vi "VISA Query.vi"(4 "VISA Timeout (0ms=Unchanged)":u32, 6 "Read Delay (0ms)":u32, 8 "error in (no error)":errorcluster, 9 "Bytes to Read (0=No read)":u32, 10 "Write (\"\"=No write)":string, 11 "VISA in":refnum<visa-resource-name>) -> (0 "error out":errorcluster, 2 "Read":string, 3 "VISA out":refnum<visa-resource-name>)   [LabVIEW 2018]
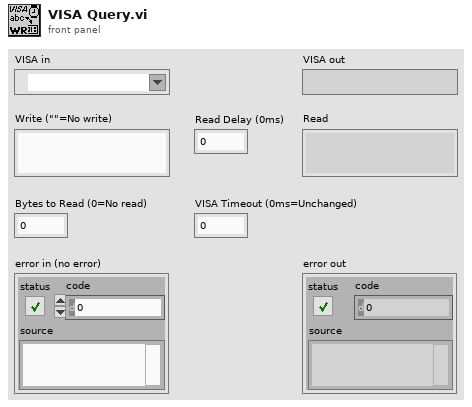
[diagram p1: front panel]
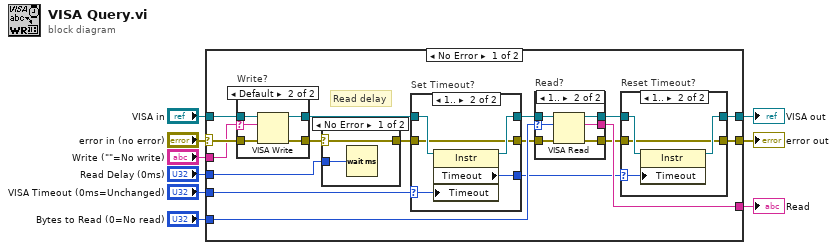
[diagram p0: block diagram]
diagram:
  n1 = case shown="No Error" "error in (no error)" {
    selector: "error in (no error)" -> [w26 w59]
    tunnel: "VISA in" -> [w25 w58]
    tunnel: "Write (\"\"=No write)" -> [w24 _]
    tunnel: "Bytes to Read (0=No read)" -> [w23 _]
    tunnel: [w22 _] -> w5
    tunnel: "Read Delay (0ms)" -> [w21 _]
    tunnel: "VISA Timeout (0ms=Unchanged)" -> [w17 _]
    tunnel: [w15 w58] -> w2
    tunnel: [w11 w59] -> w1
    frame No Error {
      # "Read delay"
      n2 = case "Write?" shown="Default" w24 {
        selector: w24 -> [_ w32]
        tunnel: w26 -> [w30 w36]
        tunnel: [w30 w35] -> w20
        tunnel: w25 -> [w31 w34]
        tunnel: [w31 w33] -> w19
        frame "" {
        }
        frame Default {
          n3 = VISA Write(VISA resource name=w34, write buffer=w32, error in (no error)=w36) -> (VISA resource name out=w33:refnum<visa-resource-name>, error out=w35:errorcluster)  [unwired: 1 out]
        }
      }
      n4 = case shown="No Error" w20 {
        selector: w20 -> [w27 w29]
        tunnel: w21 -> [w28 _]
        tunnel: [w27 w29] -> w12
        frame No Error {
          n5 = Wait (ms)(milliseconds to wait=w28) -> ()  [unwired: 1 out]
        }
        frame Error {
        }
      }
      n6 = case "Set Timeout?" shown="1.." w17 {
        selector: w17 -> [_ w41]
        tunnel: w19 -> [w38 w43]
        tunnel: [w38 w42] -> w18
        tunnel: [_ w40] -> w14
        tunnel: [w37 w39] -> w13
        tunnel: w12 -> [w37 w39]
        frame 0 {
        }
        frame 1.. {
          n7 = property class="Instr"(reference=w43, "Timeout"=w41) -> (reference out=w42:refnum<visa-resource-name>, "Timeout"=w40:u32)  [unwired: 1 in, 1 out]
        }
      }
      n8 = case "Read?" shown="1.." w23 {
        selector: w23 -> [_ w53]
        tunnel: w13 -> [w50 w57]
        tunnel: [w50 w56] -> w10
        tunnel: w18 -> [w51 w55]
        tunnel: [w51 w54] -> w16
        tunnel: [_ w52] -> w22
        frame 0 {
        }
        frame 1.. {
          n9 = VISA Read(VISA resource name=w55, byte count=w53, error in (no error)=w57) -> (VISA resource name out=w54:refnum<visa-resource-name>, read buffer=w52:string, error out=w56:errorcluster)  [unwired: 1 out]
        }
      }
      n10 = case "Reset Timeout?" shown="1.." w14 {
        selector: w14 -> [_ w47]
        tunnel: w16 -> [w45 w49]
        tunnel: [w45 w48] -> w15
        tunnel: [w44 w46] -> w11
        tunnel: w10 -> [w44 w46]
        frame 0 {
        }
        frame 1.. {
          n11 = property class="Instr"(reference=w49, "Timeout"=w47) -> (reference out=w48:refnum<visa-resource-name>)  [unwired: 1 in, 1 out]
        }
      }
    }
    frame Error {
    }
  }
  "VISA out" <- w2
  "error out" <- w1
  "Read" <- w5
